vi "HW.vi"() -> ()   [LabVIEW 2013]
panel:
  out "Grade":i32(knob) scale=0.0..100.0
  in  "Turn on":bool
  out "Rango 91-100":bool
  out "Rango 81-90":bool
  out "Rango 60-80":bool
  out "Rango 1-59":bool
  out "Rango 91-100 Sobresaliente":dbl
  out "Rango 81-90 Muy bueno":dbl
  out "Rango 60-80 Bueno":dbl
  out "Rango 1-59 Reprobado":dbl
  # "GENERAR LA NOTA DE 10 ALUMNOS, LUEGO IR CONTANDO CUANTOS ALUMNOS ESTAN EN LOS SIGUIENTES \nRANGOS:\n1-59 REPOBRADO\n60-80 BUENO\n81-90 MUY BUENO\n91-100 SOBRESALIENTE\n\nENCENDER UN LED POR CADA UNO DE LOS RANGOS"
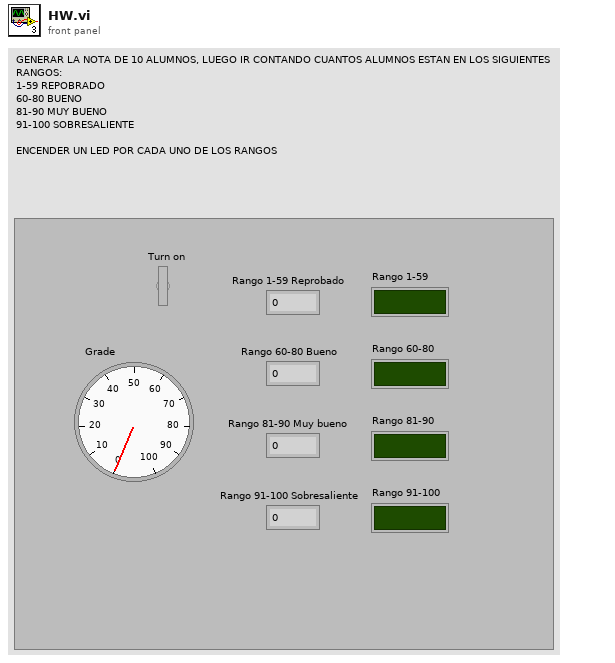
[diagram p1: front panel]
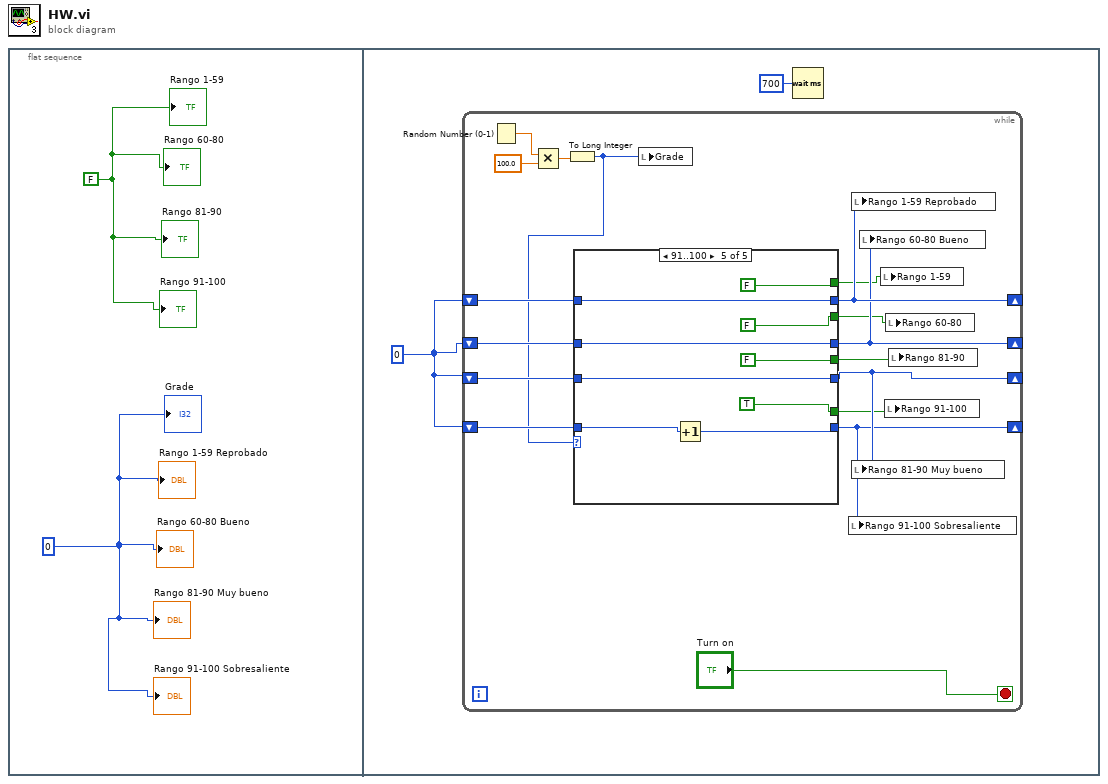
[diagram p0: block diagram]
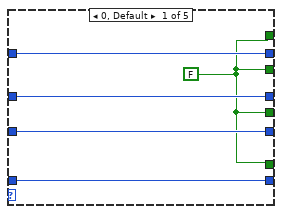
[diagram p2: hidden frame]
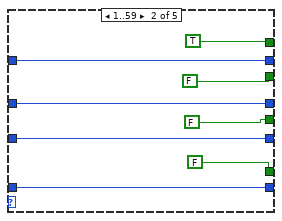
[diagram p3: hidden frame]
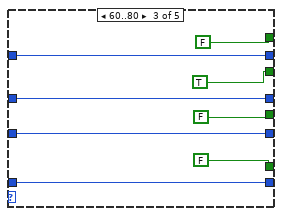
[diagram p4: hidden frame]
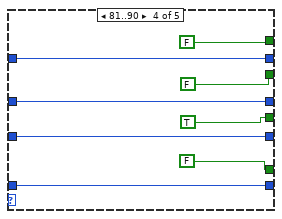
[diagram p5: hidden frame]
diagram:
  n1 = flat-sequence {
    frame #0 {
      w1 = 0 ("Nota_Alumno")
      w2 = FALSE
      "Rango 1-59" <- w2
      "Rango 81-90" <- w2
      "Rango 91-100" <- w2
      "Rango 60-80" <- w2
      "Rango 1-59 Reprobado" <- w1
      "Rango 60-80 Bueno" <- w1
      "Rango 81-90 Muy bueno" <- w1
      "Rango 91-100 Sobresaliente" <- w1
      "Grade" <- w1
    }
    frame #1 {
      w4 = 0
      n2 = while {
        shift-right: [w14] -> _
        shift-left: w4 -> [w18]
        shift-right: [w13] -> _
        shift-left: w4 -> [w17]
        shift-right: [w12] -> _
        shift-left: w4 -> [w16]
        shift-right: [w11] -> _
        shift-left: w4 -> [w15]
        stop <- "Turn on" stop-if-true
        n3 = Random Number (0-1)() -> (number: 0 to 1=w21:dbl)
        n4 = Multiply(x=w21, y=100.0) -> (x*y=w19:dbl)
        n5 = To Long Integer(number=w19) -> (32bit integer=w5:i32)
        n6 = case shown="91..100" w5 {
          tunnel: w18 -> [w26 w34 w42 w50 w59]
          tunnel: [w26 w34 w42 w50 w59] -> w14
          tunnel: w17 -> [w25 w33 w41 w49 w58]
          tunnel: [w25 w33 w41 w49 w58] -> w13
          tunnel: w16 -> [w24 w32 w40 w48 w57]
          tunnel: [w24 w32 w40 w48 w57] -> w12
          tunnel: w15 -> [w23 w31 w39 w47 w56]
          tunnel: [w23 w31 w39 w47 w55] -> w11
          tunnel: [w22 TRUE FALSE FALSE FALSE] -> w7
          tunnel: [w22 FALSE TRUE FALSE FALSE] -> w8
          tunnel: [w22 FALSE FALSE TRUE FALSE] -> w9
          tunnel: [w22 FALSE FALSE FALSE TRUE] -> w10
          frame 0, Default {
            w22 = FALSE
          }
          frame 1..59 {
          }
          frame 60..80 {
          }
          frame 81..90 {
          }
          frame 91..100 {
            n7 = Increment(x=w56) -> (x+1=w55:i32)
          }
        }
        n8 = local write "Grade"(w5) -> ()
        n9 = local write "Rango 91-100 Sobresaliente"(w11) -> ()
        n10 = local write "Rango 1-59 Reprobado"(w14) -> ()
        n11 = local write "Rango 81-90 Muy bueno"(w12) -> ()
        n12 = local write "Rango 60-80 Bueno"(w13) -> ()
        n13 = local write "Rango 1-59"(w7) -> ()
        n14 = local write "Rango 91-100"(w10) -> ()
        n15 = local write "Rango 60-80"(w8) -> ()
        n16 = local write "Rango 81-90"(w9) -> ()
      }
      n17 = Wait (ms)(milliseconds to wait=u32 700) -> ()  [unwired: 1 out]
    }
  }
